vi "GetWaveformLength.vi"(3 "error in (no error)":errorcluster, 4 "Waveform Lenght Options":u16(ring) items=["Value", "Minimum", "Maximum"], 5 "Waveform Name":string, 6 "VISA resource name":refnum<visa-resource-name>) -> (0 "error out":errorcluster, 1 "Waveform Length":i32, 2 "VISA resource name out":refnum<visa-resource-name>)   [LabVIEW 2020, in "Active Technologies AWG3000.lvlib"]
uses:
  Active Technologies AWG3000.lvlib
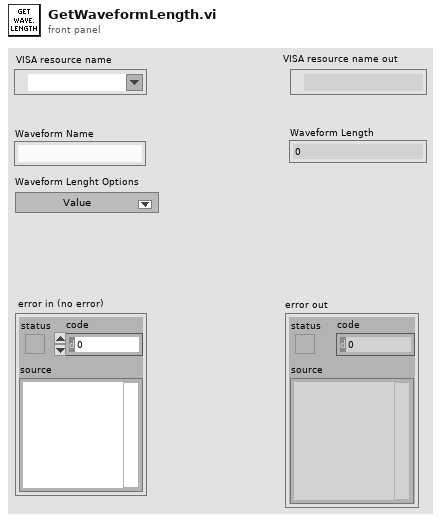
[diagram p1: front panel]
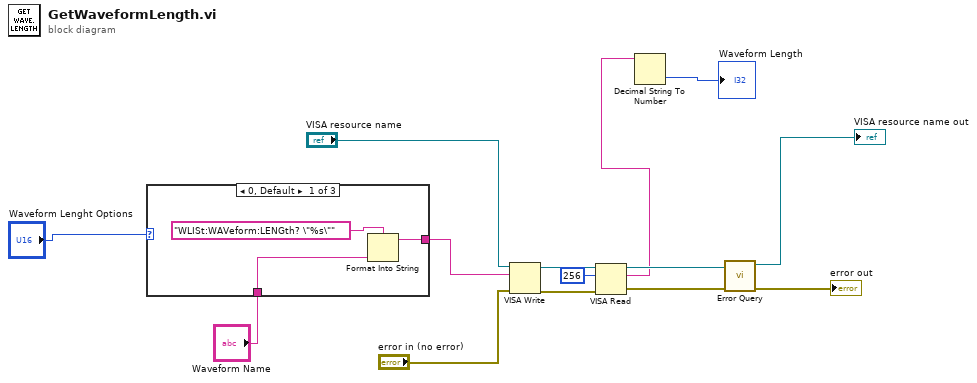
[diagram p0: block diagram]
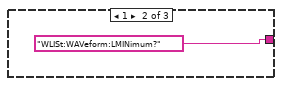
[diagram p2: hidden frame]
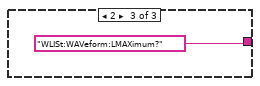
[diagram p3: hidden frame]
diagram:
  n1 = case shown="0, Default" "Waveform Lenght Options" {
    tunnel: "Waveform Name" -> [w17 _ _]
    tunnel: [w15 "WLISt:WAVeform:LMINimum?" ("write buffer") "WLISt:WAVeform:LMAXimum?" ("write buffer")] -> w3
    frame 0, Default {
      n2 = Format Into String(format string="WLISt:WAVeform:LENGth? \"%s\"" ("write buffer"), w17) -> (resulting string=w15:string)  [unwired: 2 in, 1 out]
    }
    frame 1 {
    }
    frame 2 {
    }
  }
  n3 = VISA Write(VISA resource name="VISA resource name", write buffer=w3, error in (no error)="error in (no error)") -> (VISA resource name out=w12:refnum<visa-resource-name>, error out=w11:errorcluster)  [unwired: 1 out]
  n4 = VISA Read(VISA resource name=w12, byte count=u32 256, error in (no error)=w11) -> (VISA resource name out=w9:refnum<visa-resource-name>, read buffer=w2:string, error out=w8:errorcluster)  [unwired: 1 out]
  n5 = Decimal String To Number(string=w2) -> (number=→"Waveform Length":i32)  [unwired: 2 in, 1 out]
  n6 = call "Error Query.vi"("error in (no error)"=w8, "VISA resource name"=w9) -> ("error out"=→"error out":errorcluster, "VISA resource name out"=→"VISA resource name out":refnum<visa-resource-name>)  [unwired: 6 in, 2 out]
